vi "load_FGM_data.vi"() -> (0 "H":dbl[][](array[numeric]), 1 "all rows":dbl[][](array[numeric]), 2 "Nmpc":i32, 3 "Ns":i32, 4 "M":dbl[][](array[numeric]))   [LabVIEW 2017, in "MPC_FXP_FGM_TestCase.lvclass"]
uses:
  MPC_FXP_FGM_TestCase.lvclass
  <vilib>/Utility/file.llb/Read Delimited Spreadsheet (DBL).vi
panel:
  out "size(s)":i32[](array[numeric])
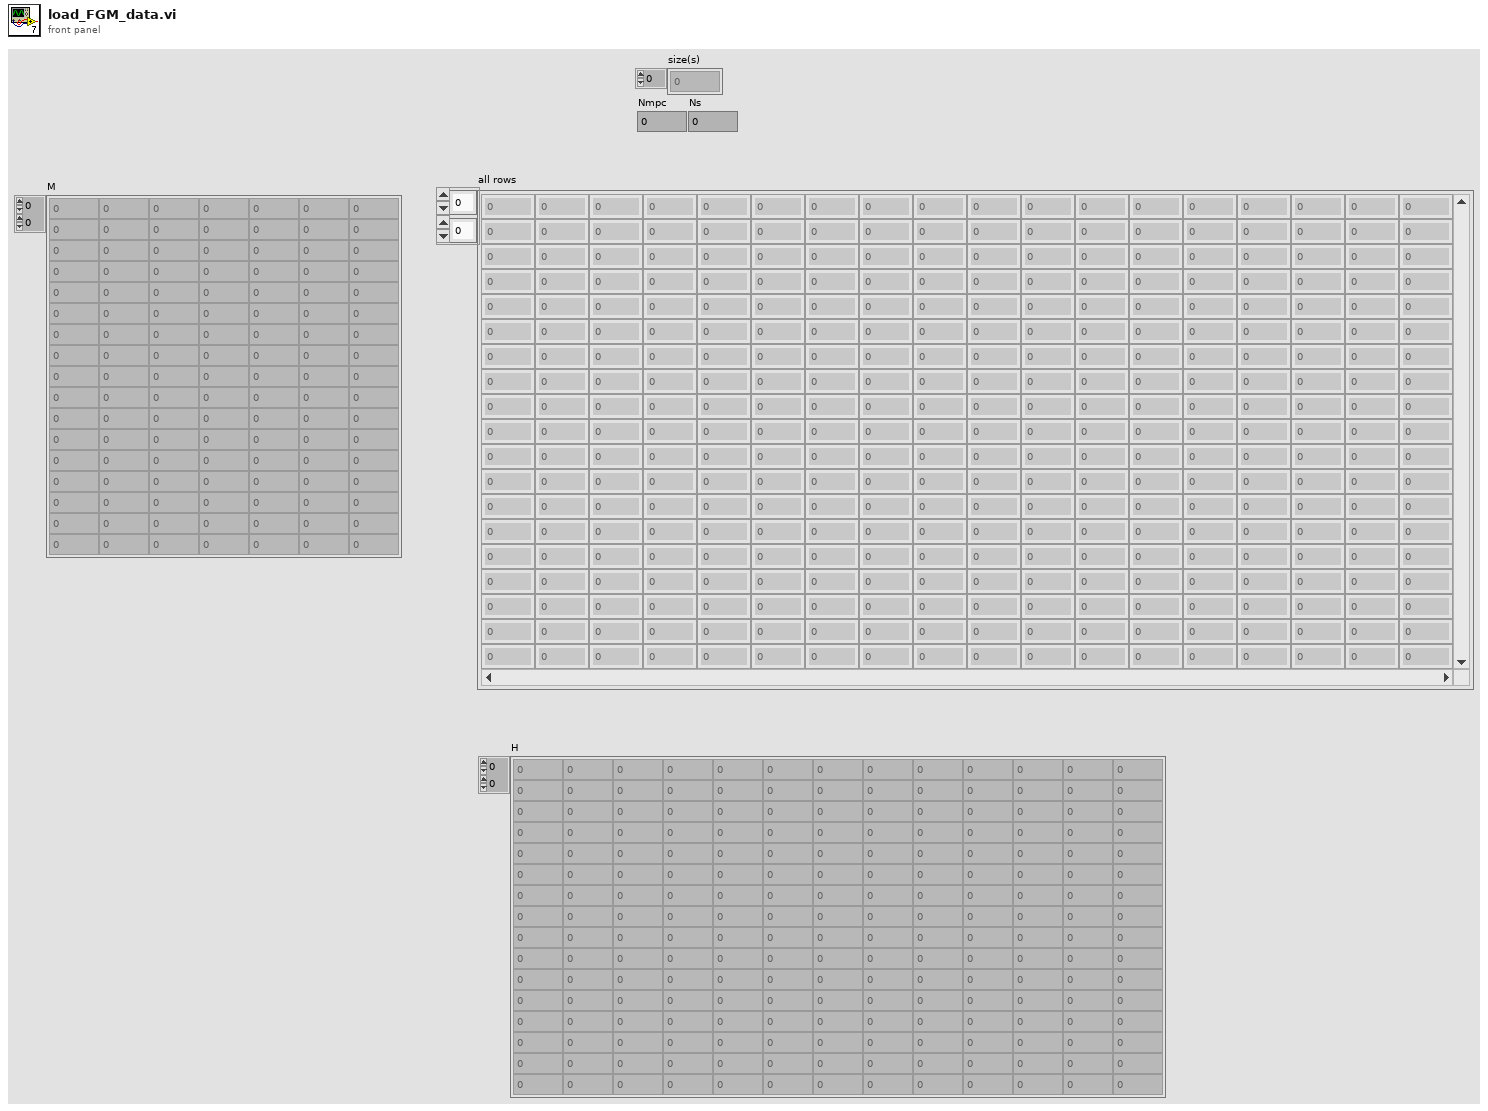
[diagram p1: front panel]
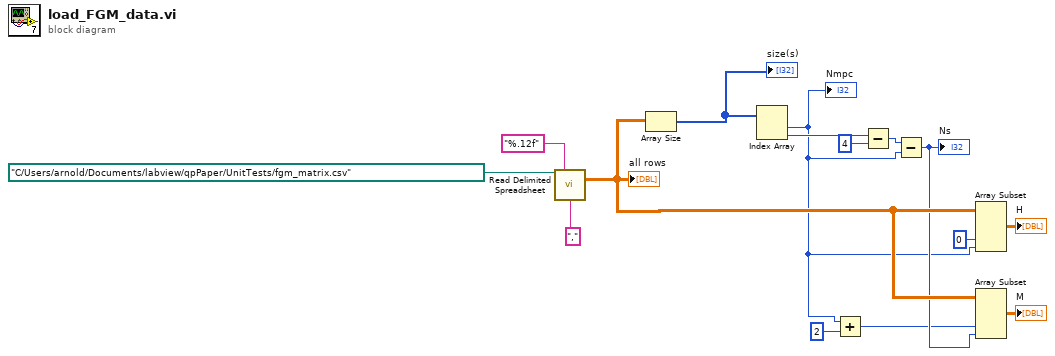
[diagram p0: block diagram]
diagram:
  n1 = call-poly <vilib>:"Read Delimited Spreadsheet.vi"("file path (dialog if empty)"=path "C:/Users/arnold/Documents/labview/qpPaper/UnitTests/fgm_matrix.csv" ("Path"), "format (%.3f)"="%.12f", "delimiter (\\t)"="," ("delimiter (\\t)")) -> ("all rows"=w7:dbl[][])  [unwired: 7 in, 5 out]
  "all rows" <- w7
  n2 = Array Size(array=w7) -> (size(s)=w12:i32[])
  "size(s)" <- w12
  n3 = Index Array(array=w12) -> (element #1=w2:i32, element #2=w11:i32)  [unwired: 2 in]
  "Nmpc" <- w2
  n4 = Add(x=w2, y=2) -> (x+y=w3:i32)
  n5 = Subtract(x=w11, y=4) -> (x-y=w9:i32)
  n6 = Subtract(x=w9, y=w2) -> (x-y=w6:i32)
  "Ns" <- w6
  n7 = Array Subset(array=w7, index (col)=0 ("index"), length (col)=w2) -> (→"H":dbl[][])  [unwired: 2 in]
  n8 = Array Subset(array=w7, index (col)=w3, length (col)=w6) -> (→"M":dbl[][])  [unwired: 2 in]
